vi "CMD_ADD.vi"(8 "error in (no error)":errorcluster, 10 "Arguments":string[](array[string]), 11 "gScript Interpreter in":refnum<class "gScript Interpreter.lvclass">) -> (0 "error out":errorcluster, 3 "gScript Interpreter out":refnum<class "gScript Interpreter.lvclass">)   [LabVIEW 2017, in "gScript Interpreter.lvclass"]
uses:
  gScript Interpreter.lvclass
  Type Definitions/Memory Cell.ctl
  Type Definitions/Memory Cell Type Enum.ctl
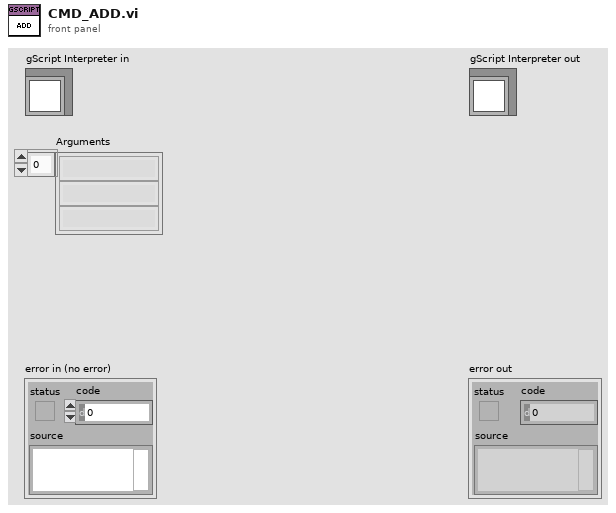
[diagram p1: front panel]
types:
  T1 = typedef "Memory Cell.ctl" = cluster{"type":T2, "x":dbl, "y":dbl, "z":dbl, "w":dbl}
  T2 = typedef "Memory Cell Type Enum.ctl" = enum16{"integer", "float", "vector", "rotation"}
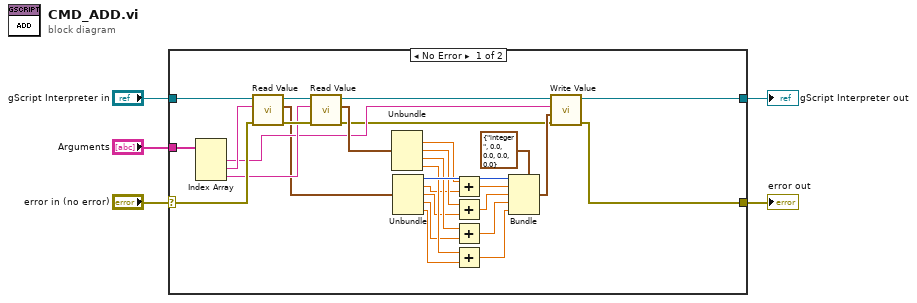
[diagram p0: block diagram]
diagram:
  n1 = case shown="No Error" "error in (no error)" {
    selector: "error in (no error)" -> [w32 w36]
    tunnel: [w6 w36] -> w4
    tunnel: [w7 w35] -> w2
    tunnel: "gScript Interpreter in" -> [w33 w35]
    tunnel: "Arguments" -> [w34 _]
    frame No Error {
      n2 = Index Array(array=w34) -> (element #1=w25:string, element #2=w31:string, element #3=w28:string)  [unwired: 3 in]
      n3 = call-dynamic "Read Value.vi"("error in (no error)"=w32, "String in"=w31, "gScript Interpreter in"=w33) -> ("error out"=w30:errorcluster, "Memory Cell"=w24:T1, "gScript Interpreter out"=w29:refnum<class "gScript Interpreter.lvclass">)  [unwired: 6 in]
      n4 = call-dynamic "Read Value.vi"("error in (no error)"=w30, "String in"=w28, "gScript Interpreter in"=w29) -> ("error out"=w21:errorcluster, "Memory Cell"=w27:T1, "gScript Interpreter out"=w26:refnum<class "gScript Interpreter.lvclass">)  [unwired: 6 in]
      n5 = Unbundle(w27) -> ("x"=w15:dbl, "y"=w14:dbl, "z"=w13:dbl, "w"=w12:dbl)  [unwired: 1 out]
      n6 = Unbundle(w24) -> ("type"=w20:T2, "x"=w11:dbl, "y"=w10:dbl, "z"=w9:dbl, "w"=w8:dbl)
      n7 = Add(x=w15, y=w11) -> (x+y=w18:dbl)
      n8 = Add(x=w14, y=w10) -> (x+y=w16:dbl)
      n9 = Add(x=w13, y=w9) -> (x+y=w17:dbl)
      n10 = Add(x=w12, y=w8) -> (x+y=w19:dbl)
      n11 = Bundle(cluster=T1 {"type"=enum."integer", "x"=0.0, "y"=0.0, "z"=0.0, "w"=0.0} ("Memory Cell"), "type"=w20, "x"=w18, "y"=w16, "z"=w17, "w"=w19) -> (w22:T1)
      n12 = call-dynamic "Write Value.vi"("error in (no error)"=w21, "Value"=w22, "Address"=w25, "gScript Interpreter in"=w26) -> ("error out"=w6:errorcluster, "gScript Interpreter out"=w7:refnum<class "gScript Interpreter.lvclass">)  [unwired: 6 in]
    }
    frame Error {
    }
  }
  "error out" <- w4
  "gScript Interpreter out" <- w2
